vi "PH_OceanOpticsSpectrometer.destructor.vi"(0 "i ref in":refnum<vi>, 5 "error in(no error)":errorcluster) -> (19 "error out":errorcluster)   [LabVIEW 2014, in "PH_OceanOpticsSpectrometer.lvlib"]
doc: "This is the destructor of a class.\n\nLicense Agreement for this software:\n\nCopyright (C)\nGesellschaft für Schwerionenforschung, GSI\nPlanckstr. 1\n64291 Darmstadt\nGermany\n\nContact: D.Beck@gsi.de \n\nThis program is free software; you can redistribute it and/or modify it under the terms of the \nGNU General Public License as published by the Free Software Foundation; either version 2 of \nthe license, or (at your option) any later version.\n\nThis program is distributed in the hope that it will be useful, but WITHOUT ANY WARRANTY; \nwithout even the implied warranty of MERCHANTABILITY or FITNESS FOR A PARTICULAR PURPOSE. See the GNU General License for more details (http://www.gnu.org).\n\nGesellschaft für Schwerionenforschung, GSI\nPlanckstr. 1, 64291 Darmstadt, Germany\nFor all questions and ideas contact: M.Richter@gsi.de, H.Brand@gsi.de or D.Beck@gsi.de.\nLast update: 16-JUN-2004"
uses:
  PH_OceanOpticsSpectrometer.lvlib
  PH_OceanOpticsSpectrometer.Trigger.ctl
  non_GPL/instr.lib/Ocean Optics 2000 4000/Ocean Optics 2000 4000 - Driver np.lvlib
  CSCore/BaseProcess/BaseProcess.lvlib
  CSCore/CSSystem/CSSystemLib/CSSystemLib.lvlib
  PH_PSDBWriter/PH_PSDBWriter.lvlib
  PH_StatusHandler/PH_StatusHandler.lvlib
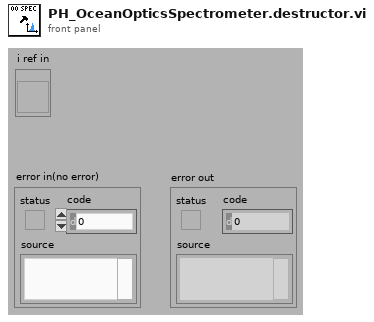
[diagram p1: front panel]
types:
  T1 = typedef "PH_OceanOpticsSpectrometer.lvlib/PH_OceanOpticsSpectrometer.Trigger.ctl" = enum32{"External", "Normal"}
  T2 = enum16{"SetAttribute", "GetAttribute", "CreateAttribute", "DestroyAttribute", "DestroyAllAtributes"}
  T3 = typedef "PH_OceanOpticsSpectrometer.lvlib/PH_OceanOpticsSpectrometer.i attribute.ctl" = cluster{"GUI Refs":cluster{"Delete":refnum<vi>, "Spectrum":refnum<vi>, "Display Width":refnum<vi>, "Display Center":refnum<vi>, "Save":refnum<vi>, "Integration time":refnum<vi>, "center wavelength":refnum<vi>, "width":refnum<vi>, "Wanted Trigger Mode":refnum<vi>, "Current Trigger Mode":refnum<vi>, "Trigger Info":refnum<vi>, "Model":refnum<vi>, "Driver":refnum<vi>, "Firmware":refnum<vi>}, "Display":cluster{"Width":dbl, "Center":dbl}, "VISA resource name":refnum<visa-resource-name>, "Integration time [ms]":cluster{"Current Value":u16, "Wanted Value":u16}, "Trigger":cluster{"Current value":T1, "Wanted value":T1}, "Default VISA Timeout":u32, "Last Data":cluster{"Wavelength Bins":dbl[], "Spectrum by Pixels":dbl[]}}
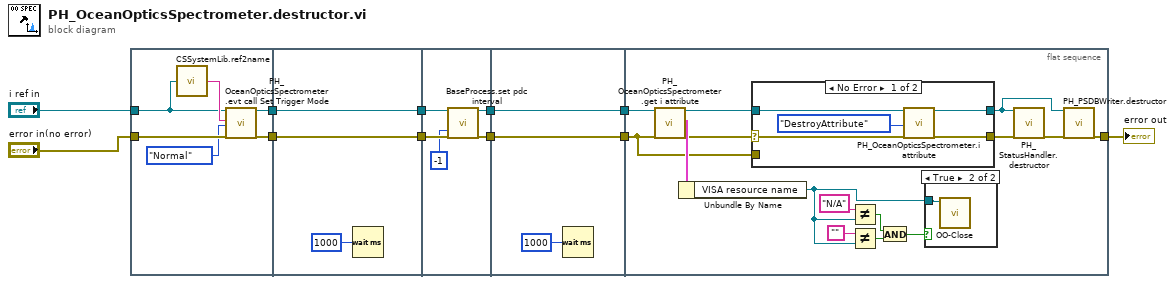
[diagram p0: block diagram]
diagram:
  n1 = flat-sequence {
    tunnel: "i ref in" -> [w15]
    tunnel: "error in(no error)" -> [w16]
    tunnel: [w13] -> w2
    tunnel: [w14] -> w1
    tunnel: [w20] -> w4
    tunnel: [w19] -> w3
    tunnel: w2 -> [w20]
    tunnel: w1 -> [w19]
    tunnel: [w22] -> w6
    tunnel: [w24] -> w5
    tunnel: w4 -> [w23]
    tunnel: w3 -> [w25]
    tunnel: [w28] -> w8
    tunnel: [w27] -> w7
    tunnel: w6 -> [w28]
    tunnel: w5 -> [w27]
    tunnel: [w33] -> w11
    tunnel: w8 -> [w29]
    tunnel: w7 -> [w42]
    frame #0 {
      n2 = call "CSSystemLib.ref2name.vi"("obj refnum"=w15) -> ("name"=w17:string)
      n3 = call "PH_OceanOpticsSpectrometer.evt call Set Trigger Mode.vi"("i ref in"=w15, "Instance"=w17, "Trigger Mode"=PH_OceanOpticsSpectrometer.Trigger."Normal", "error in (no error)"=w16) -> ("i ref out"=w14:refnum<vi>, "error out"=w13:errorcluster)  [unwired: 14 in]
    }
    frame #1 {
      n4 = Wait (ms)(milliseconds to wait=u32 1000) -> ()  [unwired: 1 out]
    }
    frame #2 {
      n5 = call "BaseProcess.set pdc interval.vi"("i ref in"=w25, "PeriodicInterval [ms]"=-1, "error in (no error)"=w23) -> ("i ref out"=w24:refnum<vi>, "error out"=w22:errorcluster)  [unwired: 14 in, 1 out]
    }
    frame #3 {
      n6 = Wait (ms)(milliseconds to wait=u32 1000) -> ()  [unwired: 1 out]
    }
    frame #4 {
      n7 = call "PH_OceanOpticsSpectrometer.get i attribute.vi"("i ref in"=w42, "error in (no error)"=w29) -> ("i ref out"=w34:refnum<vi>, "i attribute"=w41:T3, "error out"=w30:errorcluster)  [unwired: 15 in]
      n8 = Unbundle By Name(w41) -> ("VISA resource name"=w35:refnum<visa-resource-name>)
      n9 = case shown="No Error" w30 {
        selector: w30 -> [w44 _]
        tunnel: [w47 w49] -> w43
        tunnel: w34 -> [w46 w50]
        tunnel: [w45 w50] -> w31
        tunnel: w29 -> [_ w49]
        frame No Error {
          n10 = call "PH_OceanOpticsSpectrometer.i attribute.vi"("VI Refnum"=w46, "Action"=T2."DestroyAttribute", "error in (no error)"=w44) -> ("VI Refnum out"=w45:refnum<vi>, "error out"=w47:errorcluster)  [unwired: 14 in, 1 out]
        }
        frame Error {
        }
      }
      n11 = Not Equal?(x="N/A", y=w35) -> (x != y?=w39:bool)
      n12 = Not Equal?(x="", y=w35) -> (x != y?=w38:bool)
      n13 = And(x=w39, y=w38) -> (x .and. y?=w36:bool)
      n14 = case shown="True" w36 {
        tunnel: w35 -> [_ w51]
        frame False {
        }
        frame True {
          n15 = call "OO-Close.vi"("VISA resource name"=w51) -> ()  [unwired: 10 in, 1 out]
        }
      }
      n16 = call "PH_StatusHandler.destructor.vi"("i ref in"=w31, "error in(no error)"=w43) -> ("error out"=w32:errorcluster)  [unwired: 17 in]
      n17 = call "PH_PSDBWriter.destructor.vi"("i ref in"=w31, "error in(no error)"=w32) -> ("error out"=w33:errorcluster)  [unwired: 17 in]
    }
  }
  "error out" <- w11
